vi "UpdateLimsTestStepAutomation.vi"(7 "step-id":u32, 8 "error in (no error)":errorcluster, 9 "instruction automation":string, 10 "link automation":string, 11 "ByteQXAPIBase in":refnum<class "ByteQXAPIBase.lvclass">) -> (0 "error out":errorcluster, 2 "step result":T1, 3 "ByteQXAPIBase out":refnum<class "ByteQXAPIBase.lvclass">)   [LabVIEW 2019, in "ByteQXWebAPI.lvlib" / "ByteQXAPIBase.lvclass"]
doc: "Update of automation link and instruction automation data based on step-id"
uses:
  ByteQXAPIBase.lvclass
  TypeDef/UpdateLimsTestStepData.ctl
  Private/module.ctl
  ByteQXAPIBase.lvclass/ByteQXAPIBase.ctl
  <vilib>/Bytelabs/ByteREST/ByteRESTClass/ByteRESTBase/RESTBase.lvclass
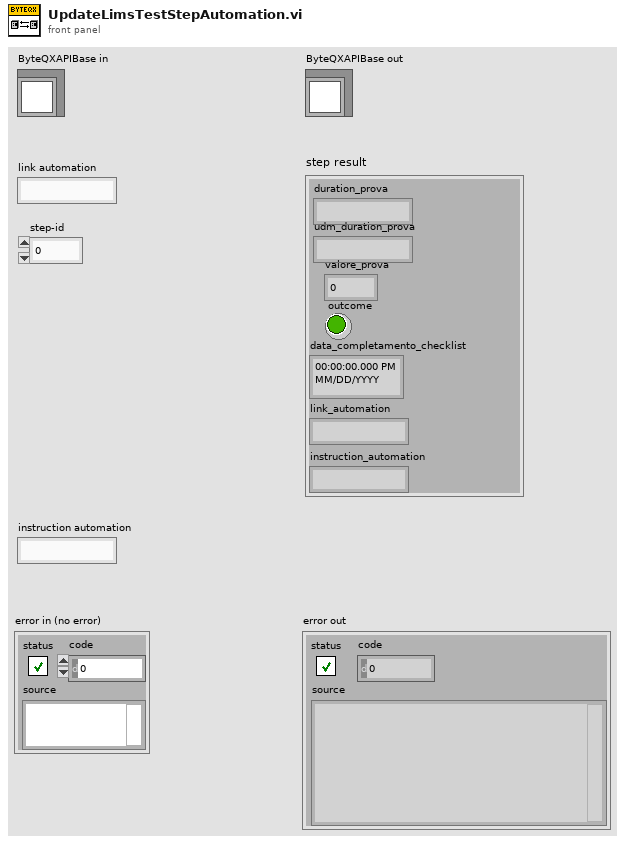
[diagram p1: front panel]
types:
  T1 = typedef "ByteQXWebAPI.lvlib/ByteQXAPIBase.lvclass/UpdateLimsTestStepData.ctl" = cluster{"outcome":bool, "data_completamento_checklist":timestamp, "udm_duration_prova":string, "valore_prova":dbl, "link_automation":string, "instruction_automation":string, "duration_prova":string}
  T2 = typedef "ByteQXWebAPI.lvlib/ByteQXAPIBase.lvclass/module.ctl" = enum16{"gs", "tms"}
  T3 = cluster{"link_automation":string, "instruction_automation":string, "udm_duration_prova":string, "outcome":string}
  T4 = cluster{"duration_prova":string, "udm_duration_prova":string, "data_completamento_checklist":string, "valore_prova":dbl, "outcome":string, "link_automation":string, "instruction_automation":string}
  T5 = typedef "ByteQXWebAPI.lvlib/ByteQXAPIBase.lvclass/Step.ctl" = cluster{"id":i32, "descrizione":string, "prova":cluster{"slug":string}, "assets":T6[], "criterio_accettazione":string, "valore_criterio_accettazione_max":dbl, "valore_criterio_accettazione_min":dbl, "udm_criterio_accettazione":string, "duration_prova":string, "udm_duration_prova":string, "valore_prova":dbl, "ordine":i32, "user":i32, "link_automation":string, "instruction_automation":string, "data_completamento_checklist":timestamp, "outcome":bool, "step_type":string, "channels":string[]}
  T6 = typedef "ByteQXWebAPI.lvlib/ByteQXAPIBase.lvclass/Asset.ctl" = cluster{"descrizione":string, "slug":string, "id":i32}
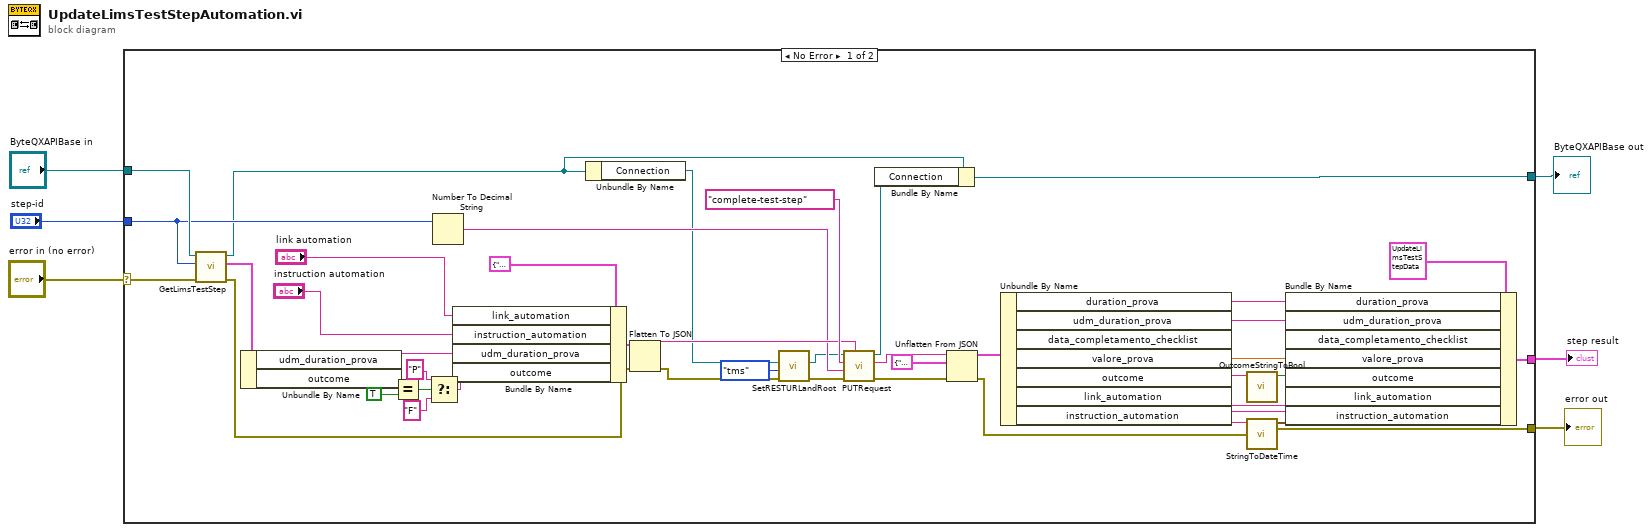
[diagram p0: block diagram]
diagram:
  n1 = case shown="No Error" "error in (no error)" {
    selector: "error in (no error)" -> [w25 w52]
    tunnel: [w37 w52] -> w5
    tunnel: [w50 w51] -> w3
    tunnel: "ByteQXAPIBase in" -> [w27 w51]
    tunnel: [w36 _] -> w2
    tunnel: "step-id" -> [w26 _]
    frame No Error {
      n2 = call-dynamic "GetLimsTestStep.vi"("error in (no error)"=w25, "step-id"=w26, "ByteQXAPIBase in"=w27) -> ("error out"=w24:errorcluster, "StepList"=w22:T5, "ByteQXAPIBase out"=w23:refnum<class "ByteQXAPIBase.lvclass">)  [unwired: 6 in]
      n3 = Unbundle By Name(w22) -> ("udm_duration_prova"=w21:string, "outcome"=w20:bool)
      n4 = Equal?(x=w20, y=TRUE) -> (x = y?=w18:bool)
      n5 = Select(t="P", s=w18, f="F") -> (s? t:f=w17:string)
      n6 = Number To Decimal String(number=w26) -> (decimal integer string=w30:string)  [unwired: 1 in]
      n7 = Bundle By Name(cluster=T3 {"link_automation"="", "instruction_automation"="", "udm_duration_prova"="", "outcome"=""}, "link_automation"="link automation", "instruction_automation"="instruction automation", "udm_duration_prova"=w21, "outcome"=w17) -> (w34:T3)
      n8 = Unbundle By Name(w23) -> ("Connection"=w9:refnum<class "RESTBase.lvclass">)
      n9 = Flatten To JSON(anything=w34, error in (no error)=w24) -> (JSON string=w47:string, 11:w11:errorcluster)  [unwired: 1 in]
      n10 = call "SetRESTURLandRoot.vi"("error in (no error)"=w11, "module"=module."tms", "ByteREST in"=w9) -> ("error out"=w10:errorcluster, "ByteREST out"=w8:refnum<class "RESTBase.lvclass">)  [unwired: 7 in]
      n11 = call-dynamic "PUTRequest.vi"("Body in"=w47, "error in (no error)"=w10, "Parameter"=w30, "Request"="complete-test-step", "ByteRESTBase in"=w8) -> ("error out"=w45:errorcluster, "Body"=w46:string, "ByteRESTBase out"=w49:refnum<class "RESTBase.lvclass">)  [unwired: 3 in, 1 out]
      n12 = Bundle By Name(cluster=w23, "Connection"=w49) -> (w50:refnum<class "ByteQXAPIBase.lvclass">)
      n13 = Unflatten From JSON(JSON string=w46, type and defaults=T4 {"duration_prova"="", "udm_duration_prova"="", "data_completamento_checklist"="", "valore_prova"=0.0, "outcome"="P", "link_automation"="", "instruction_automation"=""}, error in (no error)=w45) -> (value=w43:T4, error out=w33:errorcluster)  [unwired: 4 in]
      n14 = Unbundle By Name(w43) -> ("duration_prova"=w42:string, "udm_duration_prova"=w41:string, "data_completamento_checklist"=w39:string, "valore_prova"=w40:dbl, "outcome"=w13:string, "link_automation"=w32:string, "instruction_automation"=w31:string)
      n15 = call "OutcomeStringToBool.vi"("outcome string"=w13) -> ("outcome bool"=w12:bool)  [unwired: 10 in]
      n16 = call "StringToDateTime.vi"("error in (no error)"=w33, "datetime string"=w39) -> ("error out"=w37:errorcluster, "timestamp"=w38:timestamp)  [unwired: 8 in]
      n17 = Bundle By Name(cluster=T1 {"outcome"=FALSE, "data_completamento_checklist"=timestamp(0 s since 1904-01-01), "udm_duration_prova"="", "valore_prova"=0.0, "link_automation"="", "instruction_automation"="", "duration_prova"=""} ("Result Step"), "duration_prova"=w42, "udm_duration_prova"=w41, "data_completamento_checklist"=w38, "valore_prova"=w40, "outcome"=w12, "link_automation"=w32, "instruction_automation"=w31) -> (w36:T1)
    }
    frame Error {
    }
  }
  "error out" <- w5
  "ByteQXAPIBase out" <- w3
  "step result" <- w2
